vi "Two Mice Test.vi"() -> ()   [LabVIEW 2011]
uses:
  <vilib>/Platform/TimedLoop/XDataNode/timing_clust.ctl
  <vilib>/Platform/TimedLoop/XDataNode/nitl_modes.ctl
  <vilib>/Platform/TimedLoop/XDataNode/wakeup.ctl
  <vilib>/Platform/TimedLoop/XDataNode/XDataNode.xnode
  <vilib>/Platform/TimedLoop/XDataNode/XDNodeRunTimeDep.lvlib
panel:
  in  "Post Extraction Limit":cluster{dbl, dbl}(slide)={0.0, 6291.456} scale=-3000.0..3000.0
  in  "Distance to Camera Visible":cluster{dbl, dbl}(slide)={0.0, 6291.456} scale=-32768.0..32768.0
  out "Frame Display":T1(plugin-control)
  in  "stop":bool
  out "Image":T1(plugin-control)
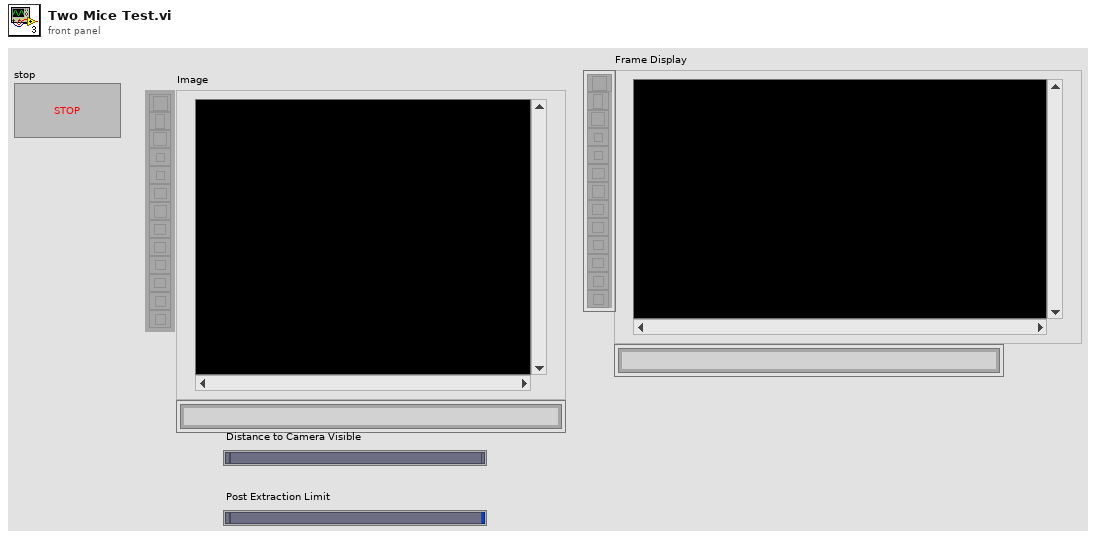
[diagram p1: front panel]
types:
  T1 = typedef "IMAQ Image.ctl" = refnum<image>
  T2 = typedef "XDNodeRunTimeDep.lvlib/timing_clust.ctl" = cluster{"Expected End [f-1]":u64, "Actual End [f-1]":u64, "Finished Late? [f-1]":bool, "Expected End [i-1]":u64, "Actual End [i-1]":u64, "Finished Late? [i-1]":bool, "Expected Start [i]":u64, "Actual Start [i]":u64, "Expected Start [f]":u64, "Actual Start [f]":u64, "Source Name":string, "Structure Name":string, "Period":i64, "Deadline":i64, "Offset":i64, "Start":i64, "Priority":i32, "Timeout":i32, "Mode":T3, "Wakeup Reason":T4, "Error":errorcluster, "Source Type":string, "Secondary Source Type":string, "Global End Time":u64, "Global Start Time":u64, "Frame Duration":u64, "Iteration Duration":u64, "Assigned CPU":i32, "I/O Scan Engine Mode":u32}
  T3 = typedef "XDNodeRunTimeDep.lvlib/nitl_modes.ctl" = enum32{"No Change", "Process missed periods, maintain original phase", "Discard missed periods, maintain original phase", "Process missed periods, ignore original phase", "Discard missed periods, ignore original phase"}
  T4 = typedef "XDNodeRunTimeDep.lvlib/wakeup.ctl" = enum32{"Normal", "Aborted", "Asynchronous wakeup", "Timing source error", "Timed loop error", "Timeout"}
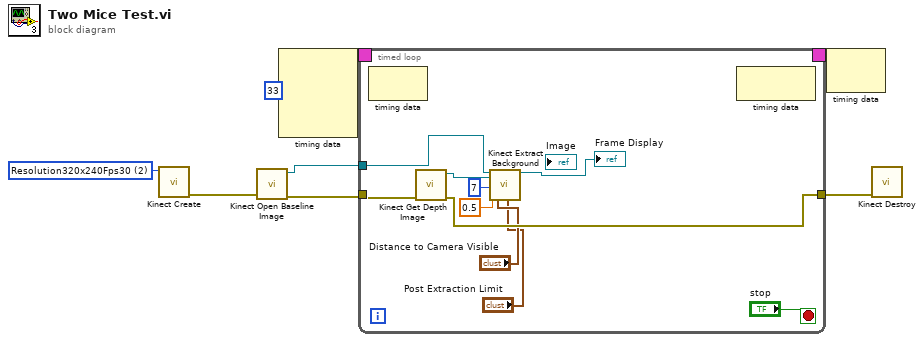
[diagram p0: block diagram]
diagram:
  w6 = 2 items=["Undefined", "Resolution640x480Fps30", "Resolution320x240Fps30", "Resolution80x60Fps30"] ("Depth Format")
  n1 = call "Kinect Create.vi"("Depth Format"=w6) -> ("error out"=w3:errorcluster)  [unwired: 10 in]
  n2 = call "Kinect Open Baseline Image.vi"("error in (no error)"=w3) -> ("error out"=w2:errorcluster, "Image Out"=w1:T1)  [unwired: 8 in, 1 out]
  n3 = node-c288(i64 33 ("Period")) -> (w8:T2)  [unwired: 3 in]
  n4 = timed-loop {
    tunnel: [w16] -> w5
    tunnel: w2 -> [w17]
    timing: w8 -> [_]
    timing-out: [_] -> w7
    tunnel: w1 -> [w15]
    stop <- "stop" stop-if-true
    n5 = node-c288() -> ()  [unwired: 1 in, 1 out]
    n6 = call "Kinect Get Depth Image.vi"("error in (no error)"=w17) -> ("error out"=w16:errorcluster, "Depth Image"=w14:T1)  [unwired: 9 in]
    n7 = call "Kinect Extract Background.vi"("Background Image In"=w15, "Depth Image In"=w14, "Median Filter Size"=7, "Divisor"=sgl 0.5, "Distance to Camera Visible"="Distance to Camera Visible", "Post Proc Bounds"="Post Extraction Limit") -> ("Processed Image Out"=→"Frame Display":T1)  [unwired: 11 in, 2 out]
    n8 = node-c288() -> ()  [unwired: 1 in, 1 out]
  }
  n9 = node-c288(w7) -> ()  [unwired: 1 out]
  n10 = call "Kinect Destroy.vi"("error in"=w5) -> ()  [unwired: 10 in, 1 out]
